vi "Device Connections.vi"(8 "error in":errorcluster, 11 "Class Objects In":T1) -> (0 "error out":errorcluster, 3 "Class Objects Out":T1)   [LabVIEW 2011]
uses:
  Controls/Class Objects.ctl
  Modules/File/Configuration/Configuration.lvclass
  Modules/Hardware/Mass Flow Controller/Mass Flow Controller.lvclass
  Modules/Hardware/Valve Controller/Valve Controller.lvclass
  Modules/Hardware/PID/PID.lvclass
  Modules/Hardware/Power Supply/Power Supply.lvclass
  Modules/Hardware/Multimeter/Multimeter.lvclass
  Modules/Hardware/Vapour Generator/Vapour Generator.lvclass
  Modules/File/TDMS/TDMS.lvclass
  Controls/Detector Type.ctl
  Controls/PS Type.ctl
  Controls/MFC Type.ctl
  Controls/Valve Type.ctl
  Modules/Hardware/Aalborg GFC17/Aalborg GFC17 Connections.ctl
  Controls/Multimeter Type.ctl
  Modules/Hardware/Owlstone GEN-SYS/GEN-SYS Connections.ctl
  Controls/Vapour Generator Type.ctl
  Modules/Hardware/Baseline Mocon piD-Tech plus/Connections.ctl
  Controls/INL PID Connections.ctl
  Modules/Hardware/INL PID/Integrator DAQmx Channels.ctl
  Functional Global Data/Device Params Global.ctl
  Controls/Class Labels.ctl
  Controls/User Interface Action.ctl
  Modules/Hardware/Aalborg GFC17/Aalborg GFC17.lvclass
  Modules/Hardware/Owlstone GEN-SYS/Owlstone GEN-SYS.lvclass
  Modules/Hardware/Baseline Mocon piD-Tech plus/Baseline Mocon piD-Tech plus.lvclass
  Modules/Hardware/INL PID/INL PID.lvclass
panel:
  in  "?":T2(tab)=enum."PID"
  in  "Vapour Generator Type":T3
  in  "Owlstone Gen-SYS":T4={"GEN-SYS VISA resource name"="", "OVG-4"={"Flow Address"=2, "Temp Address"=1}, "OHG-4"={"Flow Address"=2, "Easydew VISA resource name"=""}}
  in  "Vapour Generator Connection":bool caption="Connection"
  in  "INL PID Connections":T5={"PIDs"=1, "Integrator DAQ Channels 1"={"V0"="cDAQ1Mod1/ai0", "S1"="cDAQ1Mod5/port0/line4", "S2"="cDAQ1Mod5/ctr0"}, "Integrator DAQ Channels 2"={"V0"="cDAQ1Mod1/ai0", "S1"="cDAQ1Mod5/port0/line4", "S2"="cDAQ1Mod5/ctr0"}} {"PIDs" min=1 max=2 step=1}
  in  "B-M PID Connections":T7 caption="Baseline-Mocon piD-TECH plus"
  in  "Detector Type":T8 caption="Type"
  in  "Detector Connection":bool=TRUE caption="Connection"
  in  "Power Supply Type":T9 caption="Type"
  in  "Power Supply Connection":bool caption="Connection"
  in  "Power Supply VISA resource name":refnum<visa-resource-name> caption="VISA resource name"
  in  "Multimeter VISA resource name":refnum<visa-resource-name> caption="VISA resource name"
  in  "Multimeter Connection":bool caption="Connection"
  in  "Multimeter Type":T10 caption="Type"
  in  "Aalborg GFC17 Connections":T11={"flow rate setpoint channel"="cDAQ1Mod3/ao0", "flow rate reading channel"="cDAQ1Mod1/ai4", "valve channel"="cDAQ1Mod3/ao1"}
  in  "MFC Type":T12 caption="Type"
  in  "MFC Connection":bool=TRUE caption="Connection"
  in  "Valve Type":T13 caption="Type"
  in  "Valve Connection":bool caption="Connection"
  in  "Valve Controller VISA resource name":refnum<visa-resource-name> caption="VISA resource name"
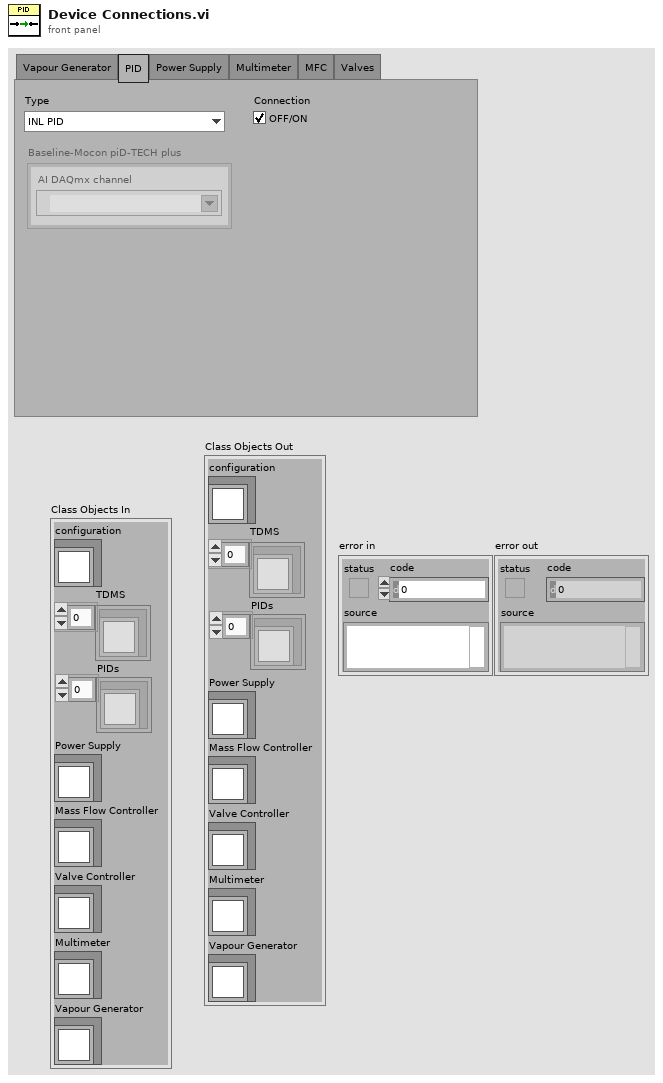
[diagram p1: front panel]
types:
  T1 = typedef "Class Objects.ctl" = cluster{"configuration":refnum<class "Configuration.lvclass">, "TDMS":refnum<class "TDMS.lvclass">[], "Power Supply":refnum<class "Power Supply.lvclass">, "Mass Flow Controller":refnum<class "Mass Flow Controller.lvclass">, "Valve Controller":refnum<class "Valve Controller.lvclass">, "Multimeter":refnum<class "Multimeter.lvclass">, "Vapour Generator":refnum<class "Vapour Generator.lvclass">, "PIDs":refnum<class "PID.lvclass">[]}
  T2 = enum32{"Vapour Generator", "PID", "Power Supply", "Multimeter", "MFC", "Valves"}
  T3 = typedef "Vapour Generator Type.ctl" = enum16{"Owlstone GEN-SYS"}
  T4 = typedef "Owlstone GEN-SYS.lvclass/GEN-SYS Connections.ctl" = cluster{"GEN-SYS VISA resource name":refnum<visa-resource-name>, "OVG-4":cluster{"Flow Address":u8, "Temp Address":u8}, "OHG-4":cluster{"Flow Address":u8, "Easydew VISA resource name":refnum<visa-resource-name>}}
  T5 = typedef "INL PID Connections.ctl" = cluster{"PIDs":u8, "Integrator DAQ Channels 1":T6, "Integrator DAQ Channels 2":T6}
  T6 = typedef "INL PID.lvclass/Integrator DAQmx Channels.ctl" = cluster{"V0":tag, "S1":tag, "S2":tag}
  T7 = typedef "Baseline Mocon piD-Tech plus.lvclass/Connections.ctl" = cluster{"AI DAQmx channel":tag}
  T8 = typedef "Detector Type.ctl" = enum16{"INL PID", "Baseline-Mocon piD-TECH plus"}
  T9 = typedef "PS Type.ctl" = enum16{"Stanford Research PS350", "Keithley 2400"}
  T10 = typedef "Multimeter Type.ctl" = enum16{"Agilent 3458A"}
  T11 = typedef "Aalborg GFC17.lvclass/Aalborg GFC17 Connections.ctl" = cluster{"flow rate setpoint channel":tag, "flow rate reading channel":tag, "valve channel":tag}
  T12 = typedef "MFC Type.ctl" = enum16{"Aalborg GFC17"}
  T13 = typedef "Valve Type.ctl" = enum16{"SMC - INL"}
  T14 = enum8{"Enabled", "Disabled", "Disabled and Grayed Out"}
  T15 = typedef "Device Params Global.ctl" = enum16{"Initialize", "Get Device Settings", "Get Device Connections", "Set Device Settings", "Set Device Connections", "Get All Device Properties"}
  T16 = typedef "Class Labels.ctl" = enum16{"Configuration", "TDMS", "PID", "Power Supply", "Vapour Generator", "MFC", "NMR", "Valve Controller", "Multimeter"}
  T17 = typedef "User Interface Action.ctl" = enum16{"Initialize", "Data Acquisition Disable", "Data View Disable", "Sample Set", "Sample Set 2D Data", "Sample Set x0 & dx", "Sample Add", "Sample Set Cursor", "Sample Set Offset & Multiplier", "Sample Set Axis Labels", "Sample Parameters Disabled", "Sample Parameters Update", "Run Update", "Run Set Offset & Multiplier", "Run Set Axis Labels", "Run Set Cursor", "Run Set Disabled", "Run Parameters Update", "Run Parameters Disabled", "Run Number Set", "Run Number Set Range", "Run Number Set Disabled", "Sample Number Set", "Sample Number Set Range", "Notes Set Value", "Update Plot", "Set Plot Parameters", "Update Concentration Plot", "Time Set", "Clear DAQ Display", "Clear Analysis Display", "Status Bar Set", "Progress Bar Set", "Display Mode Set", "Experiment Type Set", "Analysis Plot Average Set", "Stop"}
  T18 = typedef "Device Connections.ctl" = cluster{"Detector":cluster{"Detector Type":T8, "Connection":bool, "B-M PID":T7, "INL PID Connections":T5}, "Power Supply":cluster{"Type":enum16{"Stanford Research PS350", "Keithley 2400"}, "Connection":bool, "VISA resource name":refnum<visa-resource-name>}, "Mass Flow Controller":cluster{"Type":enum16{"Aalborg GFC17"}, "Connection":bool, "Aalborg GFC17":T11}, "Valve Controller":cluster{"Type":T13, "Connection":bool, "SMC - INL":cluster{"VISA resource name":refnum<visa-resource-name>}}, "Multimeter":cluster{"Multimeter Type":T10, "Connection":bool, "VISA resource name":refnum<visa-resource-name>}, "Vapour Generator":cluster{"Type":T3, "Connection":bool, "Owlstone Gen-SYS":T4}}
  T19 = enum16{"Stanford Research PS350", "Keithley 2400"}
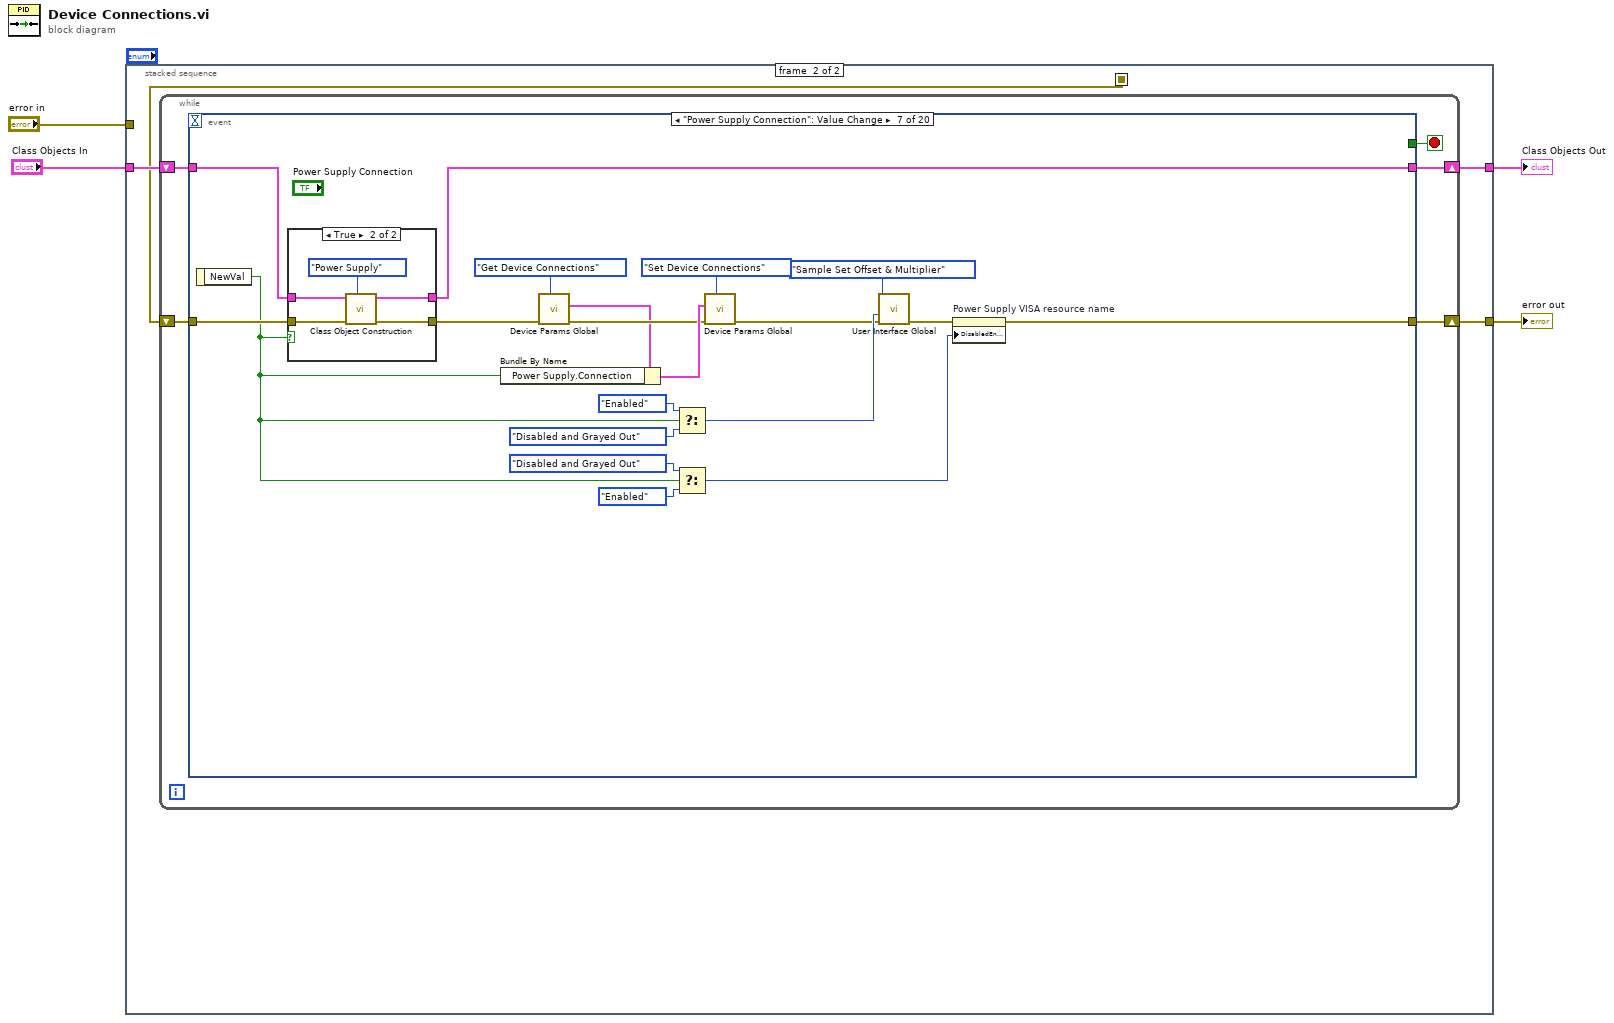
[diagram p0: block diagram]
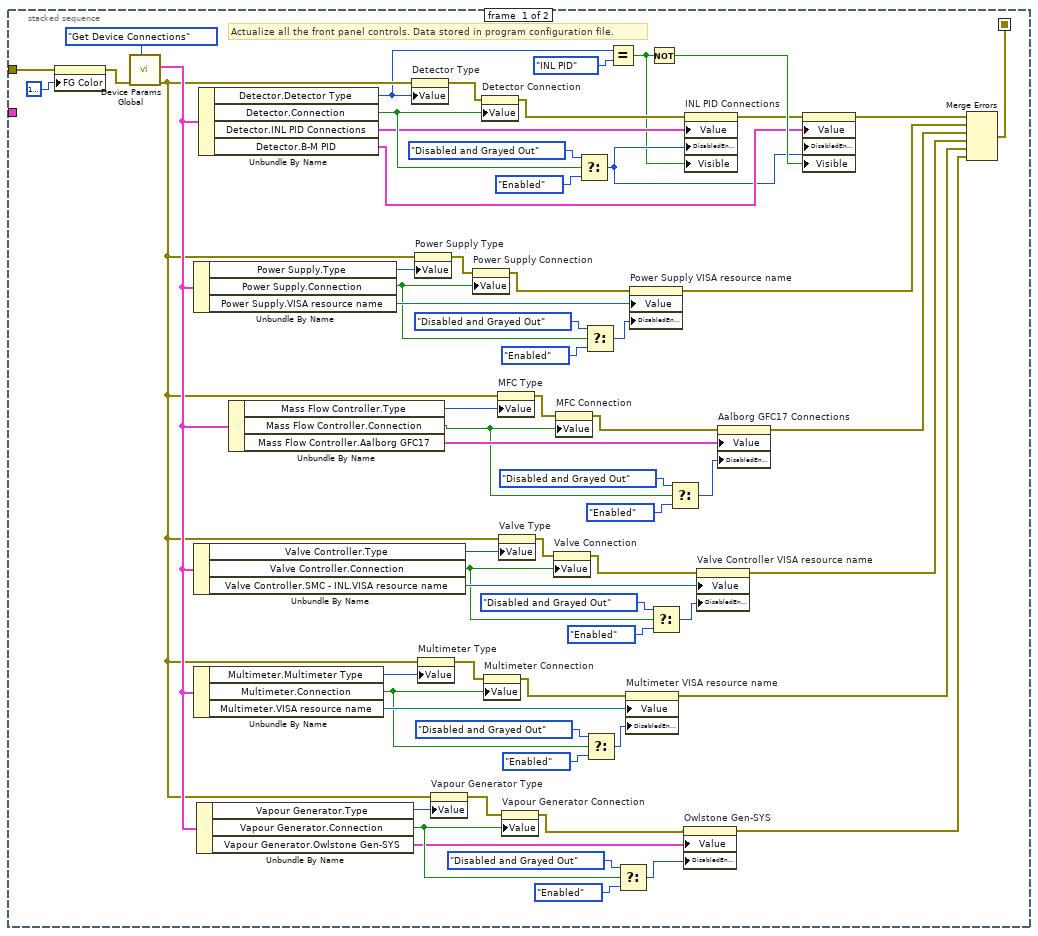
[diagram p2: hidden frame]
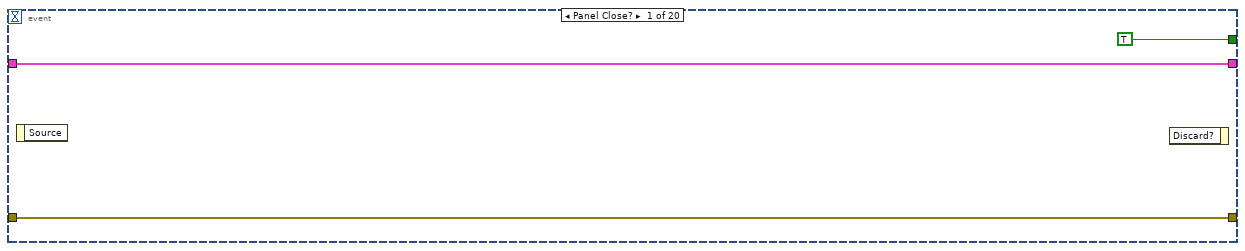
[diagram p3: hidden frame]
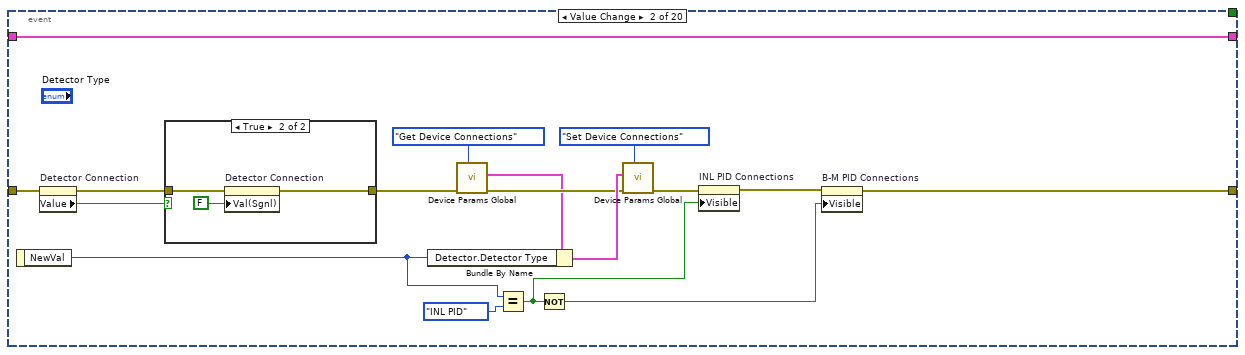
[diagram p4: hidden frame]
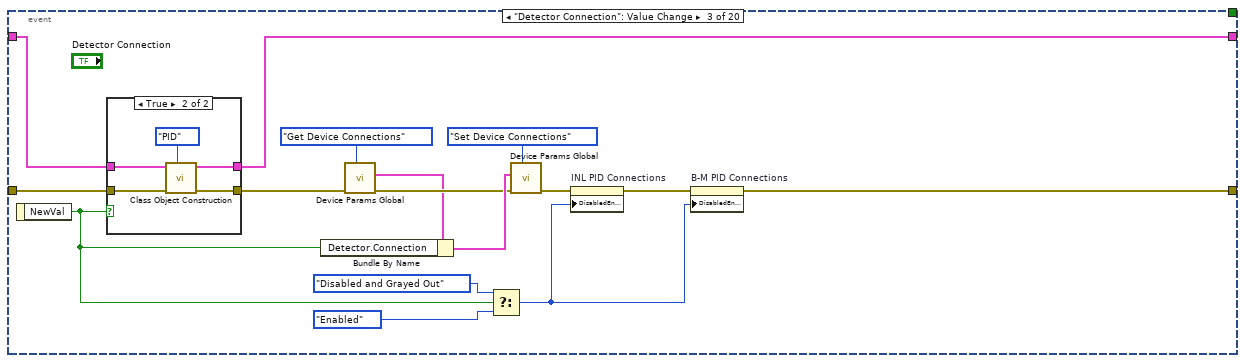
[diagram p6: hidden frame]
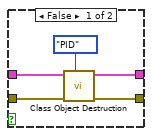
[diagram p7: hidden frame]
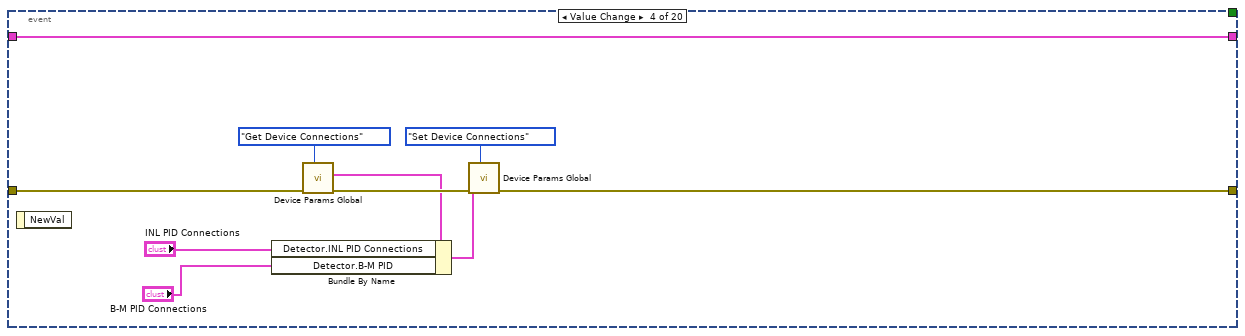
[diagram p8: hidden frame]
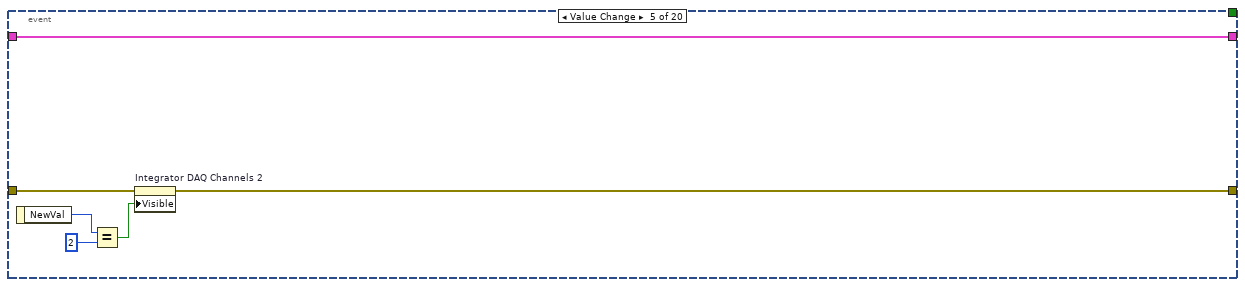
[diagram p9: hidden frame]
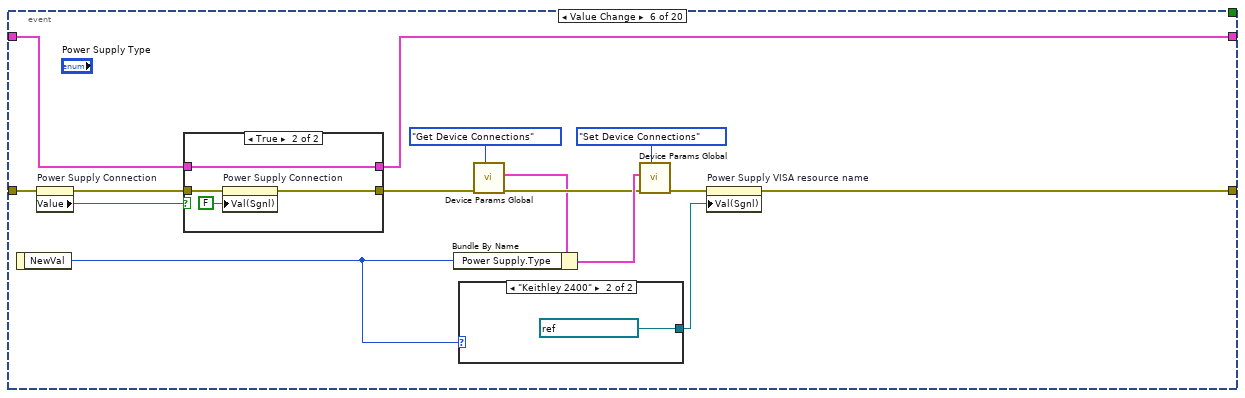
[diagram p10: hidden frame]
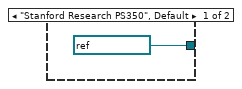
[diagram p11: hidden frame]
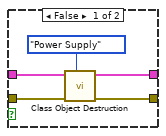
[diagram p13: hidden frame]
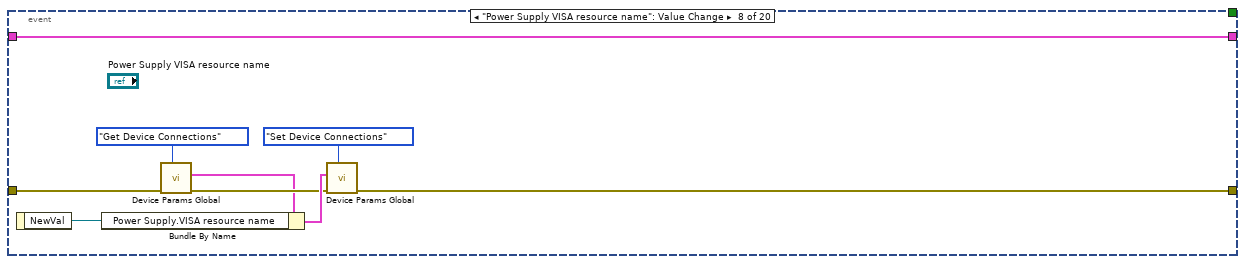
[diagram p14: hidden frame]
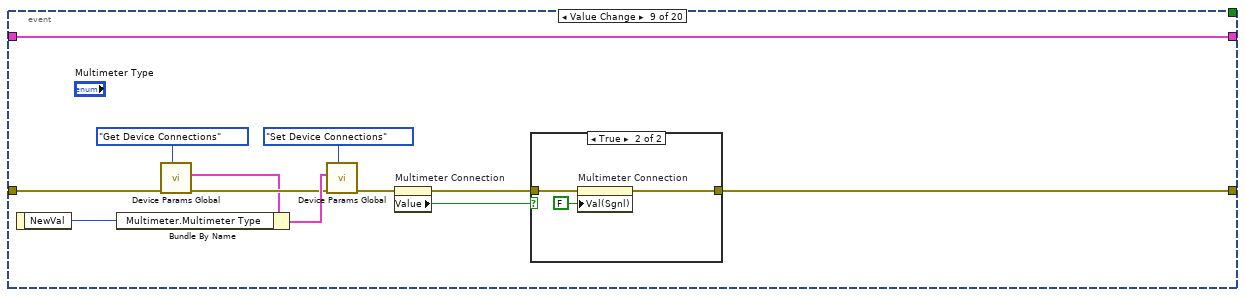
[diagram p15: hidden frame]
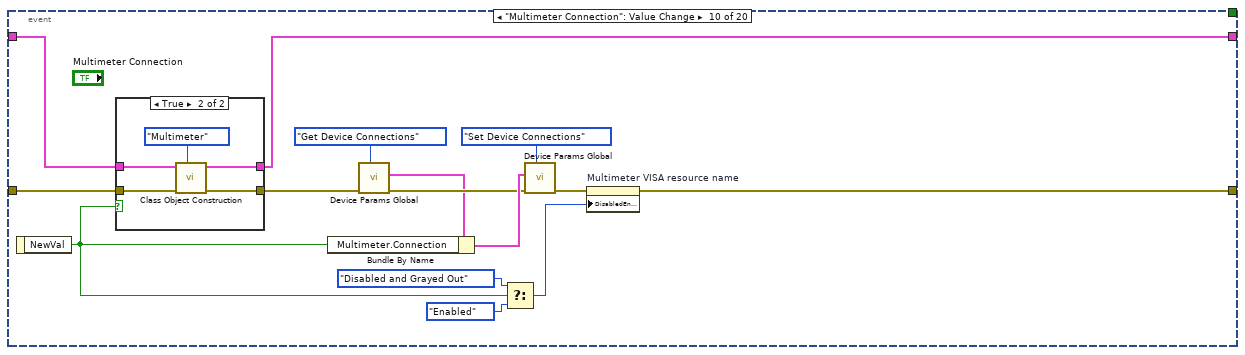
[diagram p17: hidden frame]
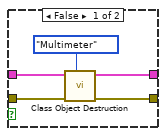
[diagram p18: hidden frame]
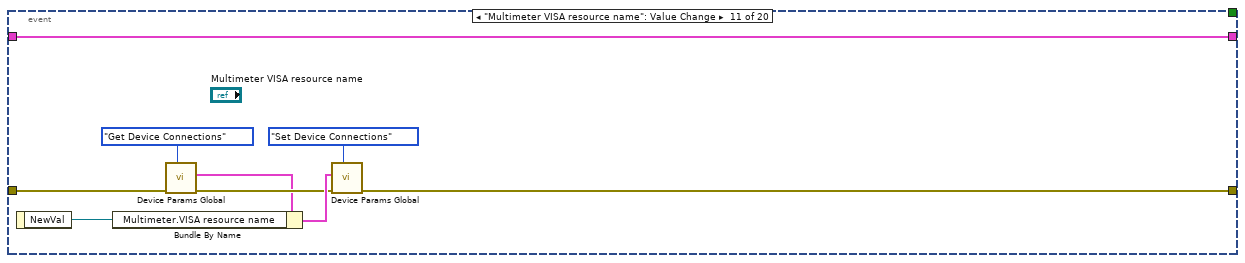
[diagram p19: hidden frame]
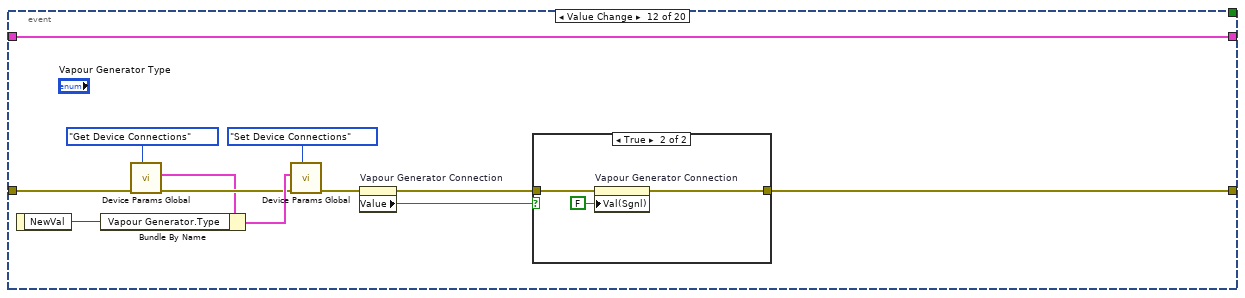
[diagram p20: hidden frame]
diagram:
  n1 = stacked-sequence {
    seq-local: [w35 _] -> [_ w71]
    tunnel: [_ w73] -> w1
    tunnel: "error in" -> [w69 _]
    tunnel: "Class Objects In" -> [_ w72]
    tunnel: [_ w74] -> w2
    frame #0 {
      # "Actualize all the front panel controls. Data stored in program configuration file."
      n2 = property class="TabCtl (strict)"(error in=w69, "FG Color"=u32 16777238) -> (error out=w68:errorcluster)  [unwired: 1 in, 1 out]
      n3 = call "Device Params Global.vi"("action"=Device_Params_Global."Get Device Connections", "error in"=w68) -> ("error out"=w16:errorcluster, "Device Connections OUT"=w25:T18)  [unwired: 7 in, 1 out]
      n4 = Unbundle By Name(w25) -> ("Power Supply.Type"=w63:T19, "Power Supply.Connection"=w46:bool, "Power Supply.VISA resource name"=w62:refnum<visa-resource-name>)
      n5 = Unbundle By Name(w25) -> ("Valve Controller.Type"=w57:T13, "Valve Controller.Connection"=w38:bool, "Valve Controller.SMC - INL.VISA resource name"=w54:refnum<visa-resource-name>)
      n6 = Unbundle By Name(w25) -> ("Multimeter.Multimeter Type"=w34:T10, "Multimeter.Connection"=w27:bool, "Multimeter.VISA resource name"=w31:refnum<visa-resource-name>)
      n7 = Unbundle By Name(w25) -> ("Vapour Generator.Type"=w15:T3, "Vapour Generator.Connection"=w22:bool, "Vapour Generator.Owlstone Gen-SYS"=w18:T4)
      n8 = Unbundle By Name(w25) -> ("Detector.Detector Type"=w12:T8, "Detector.Connection"=w50:bool, "Detector.INL PID Connections"=w7:T5, "Detector.B-M PID"=w10:T7)
      n9 = Unbundle By Name(w25) -> ("Mass Flow Controller.Type"=w61:enum16{"Aalborg GFC17"}, "Mass Flow Controller.Connection"=w42:bool, "Mass Flow Controller.Aalborg GFC17"=w58:T11)
      n10 = property on="Detector Type" class="Enum (strict)"(error in=w16, "Value"=w12) -> (error out=w66:errorcluster)  [unwired: 1 in, 1 out]
      n11 = property on="Power Supply Type" class="Enum (strict)"(error in=w16, "Value"=w63) -> (error out=w65:errorcluster)  [unwired: 1 in, 1 out]
      n12 = property on="Multimeter Type" class="Enum (strict)"(error in=w16, "Value"=w34) -> (error out=w33:errorcluster)  [unwired: 1 in, 1 out]
      n13 = property on="Vapour Generator Type" class="Enum (strict)"(error in=w16, "Value"=w15) -> (error out=w17:errorcluster)  [unwired: 1 in, 1 out]
      n14 = property on="Power Supply Connection" class="Bool (strict)"(error in=w65, "Value"=w46) -> (error out=w64:errorcluster)  [unwired: 1 in, 1 out]
      n15 = property on="Detector Connection" class="Bool (strict)"(error in=w66, "Value"=w50) -> (error out=w9:errorcluster)  [unwired: 1 in, 1 out]
      n16 = property on="Multimeter Connection" class="Bool (strict)"(error in=w33, "Value"=w27) -> (error out=w30:errorcluster)  [unwired: 1 in, 1 out]
      n17 = property on="MFC Type" class="Enum (strict)"(error in=w16, "Value"=w61) -> (error out=w60:errorcluster)  [unwired: 1 in, 1 out]
      n18 = property on="Valve Type" class="Enum (strict)"(error in=w16, "Value"=w57) -> (error out=w56:errorcluster)  [unwired: 1 in, 1 out]
      n19 = property on="Vapour Generator Connection" class="Bool (strict)"(error in=w17, "Value"=w22) -> (error out=w19:errorcluster)  [unwired: 1 in, 1 out]
      n20 = property on="Valve Connection" class="Bool (strict)"(error in=w56, "Value"=w38) -> (error out=w55:errorcluster)  [unwired: 1 in, 1 out]
      n21 = property on="MFC Connection" class="Bool (strict)"(error in=w60, "Value"=w42) -> (error out=w59:errorcluster)  [unwired: 1 in, 1 out]
      n22 = Select(t=T14."Disabled and Grayed Out" ("Disabled"), s=w50, f=T14."Enabled") -> (s? t:f=w6:T14)
      n23 = Select(t=T14."Disabled and Grayed Out" ("Disabled"), s=w46, f=T14."Enabled") -> (s? t:f=w45:T14)
      n24 = Select(t=T14."Disabled and Grayed Out" ("Disabled"), s=w27, f=T14."Enabled") -> (s? t:f=w29:T14)
      n25 = Equal?(x=w12, y=Detector_Type."INL PID" ("Detector.Detector Type")) -> (x = y?=w5:bool)
      n26 = Select(t=T14."Disabled and Grayed Out" ("Disabled"), s=w22, f=T14."Enabled") -> (s? t:f=w21:T14)
      n27 = property on="Multimeter VISA resource name" class="VISAName"(error in=w30, "Value"=w31, "DisabledEnum"=w29) -> (error out=w26:errorcluster)  [unwired: 1 in, 1 out]
      n28 = property on="Power Supply VISA resource name" class="VISAName"(error in=w64, "Value"=w62, "DisabledEnum"=w45) -> (error out=w53:errorcluster)  [unwired: 1 in, 1 out]
      n29 = Not(x=w5) -> (.not. x?=w11:bool)
      n30 = Select(t=T14."Disabled and Grayed Out" ("Disabled"), s=w38, f=T14."Enabled") -> (s? t:f=w37:T14)
      n31 = Select(t=T14."Disabled and Grayed Out" ("Disabled"), s=w42, f=T14."Enabled") -> (s? t:f=w41:T14)
      n32 = property on="Owlstone Gen-SYS" class="Clust (strict)"(error in=w19, "Value"=w18, "DisabledEnum"=w21) -> (error out=w20:errorcluster)  [unwired: 1 in, 1 out]
      n33 = property on="INL PID Connections" class="Clust (strict)"(error in=w9, "Value"=w7, "DisabledEnum"=w6, "Visible"=w5) -> (error out=w8:errorcluster)  [unwired: 1 in, 1 out]
      n34 = property on="Valve Controller VISA resource name" class="VISAName"(error in=w55, "Value"=w54, "DisabledEnum"=w37) -> (error out=w36:errorcluster)  [unwired: 1 in, 1 out]
      n35 = property on="Aalborg GFC17 Connections" class="Clust (strict)"(error in=w59, "Value"=w58, "DisabledEnum"=w41) -> (error out=w52:errorcluster)  [unwired: 1 in, 1 out]
      n36 = property on="B-M PID Connections" class="Clust (strict)"(error in=w8, "Value"=w10, "DisabledEnum"=w6, "Visible"=w11) -> (error out=w14:errorcluster)  [unwired: 1 in, 1 out]
      n37 = Merge Errors(w14, w53, w52, w36, w26, w20) -> (w35:errorcluster)
    }
    frame #1 {
      n38 = while {
        shift-right: [w77] -> w74
        shift-left: w72 -> [w78]
        shift-right: [w75] -> w73
        shift-left: w71 -> [w76]
        stop <- w79 stop-if-true
        n39 = event shown="[6] \"Power Supply Connection\": Value Change" {
          selector: _ -> [_ _ _ _ _ _ _ _ _ _ _ _ _ _ _ _ _ _ _ _]
          dyn-events: _ -> [_ _ _ _ _ _ _ _ _ _ _ _ _ _ _ _ _ _ _ _]
          timeout: _ -> [_ _ _ _ _ _ _ _ _ _ _ _ _ _ _ _ _ _ _ _]
          tunnel: [w81 w86 w107 w132 w140 w154 w183 w205 w208 w230 w250 w259 w274 w301 w316 w335 w349 w366 w381 w397] -> w75
          tunnel: [TRUE ("Discard?") _ _ _ _ _ _ _ _ _ _ _ _ _ _ _ _ _ _ _] -> w79
          tunnel: w78 -> [w82 w99 w119 w139 w143 w160 w188 w203 w219 w228 w249 w258 w288 w300 w319 w338 w357 w369 w387 w405]
          tunnel: [w82 w99 w118 w139 w143 w156 w187 w203 w219 w227 w249 w258 w277 w300 w319 w337 w357 w369 w386 w405] -> w77
          tunnel: w76 -> [w81 w98 w117 w133 w141 w159 w177 w201 w213 w229 w252 w264 w287 w302 w310 w336 w351 w360 w385 w399]
          event Panel Close? {
            n40 = event-data() -> ()  [unwired: 1 in, 1 out]
            n41 = event-data() -> ()  [unwired: 2 in, 1 out]
          }
          event Value Change {
            n42 = event-data() -> ("NewVal"=w88:T8)  [unwired: 1 in]
            n43 = property on="Detector Connection" class="Bool (strict)"(error in=w98) -> (error out=w96:errorcluster, "Value"=w97:bool)  [unwired: 1 in, 1 out]
            n44 = case shown="True" w97 {
              tunnel: w96 -> [w100 w103]
              tunnel: [w100 w102] -> w90
              frame False {
              }
              frame True {
                n45 = property on="Detector Connection" class="Bool (strict)"(error in=w103, "Val(Sgnl)"=FALSE ("Detector Connection")) -> (error out=w102:errorcluster)  [unwired: 1 in, 1 out]
              }
            }
            n46 = call "Device Params Global.vi"("action"=Device_Params_Global."Get Device Connections", "error in"=w90) -> ("error out"=w92:errorcluster, "Device Connections OUT"=w91:T18)  [unwired: 7 in, 1 out]
            n47 = Bundle By Name(cluster=w91, "Detector.Detector Type"=w88) -> (w94:T18)
            n48 = Equal?(x=w88, y=Detector_Type."INL PID" ("Detector.Detector Type")) -> (x = y?=w84:bool)
            n49 = Not(x=w84) -> (.not. x?=w87:bool)
            n50 = call "Device Params Global.vi"("action"=Device_Params_Global."Set Device Connections", "error in"=w92, "Device Connections IN"=w94) -> ("error out"=w85:errorcluster)  [unwired: 6 in, 2 out]
            n51 = property on="INL PID Connections" class="Clust (strict)"(error in=w85, "Visible"=w84) -> (error out=w83:errorcluster)  [unwired: 1 in, 1 out]
            n52 = property on="B-M PID Connections" class="Clust (strict)"(error in=w83, "Visible"=w87) -> (error out=w86:errorcluster)  [unwired: 1 in, 1 out]
          }
          event "Detector Connection": Value Change {
            n53 = event-data() -> ("NewVal"=w108:bool)  [unwired: 1 in]
            n54 = case shown="True" w108 {
              tunnel: w119 -> [w122 w129]
              tunnel: w117 -> [w124 w127]
              tunnel: [w121 w126] -> w118
              tunnel: [w123 w125] -> w109
              frame False {
                n55 = call "Class Object Destruction.vi"("class labels"=Class_Labels."PID", "error in"=w124, "classes in"=w122) -> ("error out"=w123:errorcluster, "classes out"=w121:T1)  [unwired: 7 in]
              }
              frame True {
                n56 = call "Class Object Construction.vi"("class"=Class_Labels."PID", "error in"=w127, "classes in"=w129) -> ("error out"=w125:errorcluster, "classes out"=w126:T1)  [unwired: 6 in]
              }
            }
            n57 = call "Device Params Global.vi"("action"=Device_Params_Global."Get Device Connections", "error in"=w109) -> ("error out"=w111:errorcluster, "Device Connections OUT"=w110:T18)  [unwired: 7 in, 1 out]
            n58 = Bundle By Name(cluster=w110, "Detector.Connection"=w108) -> (w113:T18)
            n59 = Select(t=T14."Disabled and Grayed Out" ("Disabled"), s=w108, f=T14."Enabled" ("Disabled")) -> (s? t:f=w105:T14)
            n60 = call "Device Params Global.vi"("action"=Device_Params_Global."Set Device Connections", "error in"=w111, "Device Connections IN"=w113) -> ("error out"=w106:errorcluster)  [unwired: 6 in, 2 out]
            n61 = property on="INL PID Connections" class="Clust (strict)"(error in=w106, "DisabledEnum"=w105) -> (error out=w104:errorcluster)  [unwired: 1 in, 1 out]
            n62 = property on="B-M PID Connections" class="Clust (strict)"(error in=w104, "DisabledEnum"=w105) -> (error out=w107:errorcluster)  [unwired: 1 in, 1 out]
          }
          event Value Change {
            n63 = event-data() -> ()  [unwired: 1 in, 1 out]
            n64 = call "Device Params Global.vi"("action"=Device_Params_Global."Get Device Connections", "error in"=w133) -> ("error out"=w135:errorcluster, "Device Connections OUT"=w134:T18)  [unwired: 7 in, 1 out]
            n65 = Bundle By Name(cluster=w134, "Detector.INL PID Connections"="INL PID Connections", "Detector.B-M PID"="B-M PID Connections") -> (w137:T18)
            n66 = call "Device Params Global.vi"("action"=Device_Params_Global."Set Device Connections", "error in"=w135, "Device Connections IN"=w137) -> ("error out"=w132:errorcluster)  [unwired: 6 in, 2 out]
          }
          event Value Change {
            n67 = event-data() -> ("NewVal"=w144:u8)  [unwired: 1 in]
            n68 = Equal?(x=w144, y=2) -> (x = y?=w142:bool)
            n69 = property on="Integrator DAQ Channels 2" class="Clust (strict)"(error in=w141, "Visible"=w142) -> (error out=w140:errorcluster)  [unwired: 1 in, 1 out]
          }
          event Value Change {
            n70 = event-data() -> ("NewVal"=w146:T9)  [unwired: 1 in]
            n71 = property on="Power Supply Connection" class="Bool (strict)"(error in=w159) -> (error out=w158:errorcluster, "Value"=w157:bool)  [unwired: 1 in, 1 out]
            n72 = case shown="True" w157 {
              tunnel: w160 -> [w164 w166]
              tunnel: [w163 w167] -> w148
              tunnel: [w164 w166] -> w156
              tunnel: w158 -> [w163 w165]
              frame False {
              }
              frame True {
                n73 = property on="Power Supply Connection" class="Bool (strict)"(error in=w165, "Val(Sgnl)"=FALSE ("PS Connection")) -> (error out=w167:errorcluster)  [unwired: 1 in, 1 out]
              }
            }
            n74 = case shown="\"Keithley 2400\"" w146 {
              tunnel: [refnum<visa-resource-name> "SR_PS350" ("VISA resource name") refnum<visa-resource-name> "Keithley_2400" ("VISA resource name")] -> w155
              frame "Stanford Research PS350", Default {
              }
              frame "Keithley 2400" {
              }
            }
            n75 = call "Device Params Global.vi"("action"=Device_Params_Global."Get Device Connections", "error in"=w148) -> ("error out"=w150:errorcluster, "Device Connections OUT"=w149:T18)  [unwired: 7 in, 1 out]
            n76 = Bundle By Name(cluster=w149, "Power Supply.Type"=w146) -> (w152:T18)
            n77 = call "Device Params Global.vi"("action"=Device_Params_Global."Set Device Connections", "error in"=w150, "Device Connections IN"=w152) -> ("error out"=w147:errorcluster)  [unwired: 6 in, 2 out]
            n78 = property on="Power Supply VISA resource name" class="VISAName"(error in=w147, "Val(Sgnl)"=w155) -> (error out=w154:errorcluster)  [unwired: 1 in, 1 out]
          }
          event "Power Supply Connection": Value Change {
            n79 = event-data() -> ("NewVal"=w169:bool)  [unwired: 1 in]
            n80 = case shown="True" w169 {
              tunnel: w188 -> [w192 w198]
              tunnel: [w191 w195] -> w187
              tunnel: [w193 w196] -> w171
              tunnel: w177 -> [w189 w197]
              frame False {
                n81 = call "Class Object Destruction.vi"("class labels"=Class_Labels."Power Supply", "error in"=w189, "classes in"=w192) -> ("error out"=w193:errorcluster, "classes out"=w191:T1)  [unwired: 7 in]
              }
              frame True {
                n82 = call "Class Object Construction.vi"("class"=Class_Labels."Power Supply", "error in"=w197, "classes in"=w198) -> ("error out"=w196:errorcluster, "classes out"=w195:T1)  [unwired: 6 in]
              }
            }
            n83 = call "Device Params Global.vi"("action"=Device_Params_Global."Get Device Connections", "error in"=w171) -> ("error out"=w173:errorcluster, "Device Connections OUT"=w172:T18)  [unwired: 7 in, 1 out]
            n84 = Bundle By Name(cluster=w172, "Power Supply.Connection"=w169) -> (w175:T18)
            n85 = Select(t=T14."Enabled" ("Disabled"), s=w169, f=T14."Disabled and Grayed Out" ("Disabled")) -> (s? t:f=w178:T14)
            n86 = Select(t=T14."Disabled and Grayed Out" ("Disabled"), s=w169, f=T14."Enabled" ("Disabled")) -> (s? t:f=w182:T14)
            n87 = call "Device Params Global.vi"("action"=Device_Params_Global."Set Device Connections", "error in"=w173, "Device Connections IN"=w175) -> ("error out"=w170:errorcluster)  [unwired: 6 in, 2 out]
            n88 = call "User Interface Global.vi"("error in"=w170, "data1"=w178, "action"=User_Interface_Action."Sample Set Offset & Multiplier") -> ("error out"=w184:errorcluster)  [unwired: 8 in]
            n89 = property on="Power Supply VISA resource name" class="VISAName"(error in=w184, "DisabledEnum"=w182) -> (error out=w183:errorcluster)  [unwired: 1 in, 1 out]
          }
          event "Power Supply VISA resource name": Value Change {
            n90 = event-data() -> ("NewVal"=w204:refnum<visa-resource-name>)  [unwired: 1 in]
            n91 = call "Device Params Global.vi"("action"=Device_Params_Global."Get Device Connections", "error in"=w201) -> ("error out"=w200:errorcluster, "Device Connections OUT"=w199:T18)  [unwired: 7 in, 1 out]
            n92 = Bundle By Name(cluster=w199, "Power Supply.VISA resource name"=w204) -> (w206:T18)
            n93 = call "Device Params Global.vi"("action"=Device_Params_Global."Set Device Connections", "error in"=w200, "Device Connections IN"=w206) -> ("error out"=w205:errorcluster)  [unwired: 6 in, 2 out]
          }
          event Value Change {
            n94 = event-data() -> ("NewVal"=w212:T10)  [unwired: 1 in]
            n95 = call "Device Params Global.vi"("action"=Device_Params_Global."Get Device Connections", "error in"=w213) -> ("error out"=w215:errorcluster, "Device Connections OUT"=w214:T18)  [unwired: 7 in, 1 out]
            n96 = Bundle By Name(cluster=w214, "Multimeter.Multimeter Type"=w212) -> (w217:T18)
            n97 = call "Device Params Global.vi"("action"=Device_Params_Global."Set Device Connections", "error in"=w215, "Device Connections IN"=w217) -> ("error out"=w211:errorcluster)  [unwired: 6 in, 2 out]
            n98 = property on="Multimeter Connection" class="Bool (strict)"(error in=w211) -> (error out=w209:errorcluster, "Value"=w210:bool)  [unwired: 1 in, 1 out]
            n99 = case shown="True" w210 {
              tunnel: w209 -> [w220 w223]
              tunnel: [w220 w221] -> w208
              frame False {
              }
              frame True {
                n100 = property on="Multimeter Connection" class="Bool (strict)"(error in=w223, "Val(Sgnl)"=FALSE ("Value (Signaling)")) -> (error out=w221:errorcluster)  [unwired: 1 in, 1 out]
              }
            }
          }
          event "Multimeter Connection": Value Change {
            n101 = event-data() -> ("NewVal"=w226:bool)  [unwired: 1 in]
            n102 = case shown="True" w226 {
              tunnel: w228 -> [w242 w248]
              tunnel: [w241 w246] -> w227
              tunnel: [w243 w245] -> w225
              tunnel: w229 -> [w239 w244]
              frame False {
                n103 = call "Class Object Destruction.vi"("class labels"=Class_Labels."Multimeter", "error in"=w239, "classes in"=w242) -> ("error out"=w243:errorcluster, "classes out"=w241:T1)  [unwired: 7 in]
              }
              frame True {
                n104 = call "Class Object Construction.vi"("class"=Class_Labels."Multimeter", "error in"=w244, "classes in"=w248) -> ("error out"=w245:errorcluster, "classes out"=w246:T1)  [unwired: 6 in]
              }
            }
            n105 = call "Device Params Global.vi"("action"=Device_Params_Global."Get Device Connections", "error in"=w225) -> ("error out"=w235:errorcluster, "Device Connections OUT"=w234:T18)  [unwired: 7 in, 1 out]
            n106 = Bundle By Name(cluster=w234, "Multimeter.Connection"=w226) -> (w237:T18)
            n107 = Select(t=T14."Disabled and Grayed Out" ("Disabled"), s=w226, f=T14."Enabled" ("Disabled")) -> (s? t:f=w231:T14)
            n108 = call "Device Params Global.vi"("action"=Device_Params_Global."Set Device Connections", "error in"=w235, "Device Connections IN"=w237) -> ("error out"=w232:errorcluster)  [unwired: 6 in, 2 out]
            n109 = property on="Multimeter VISA resource name" class="VISAName"(error in=w232, "DisabledEnum"=w231) -> (error out=w230:errorcluster)  [unwired: 1 in, 1 out]
          }
          event "Multimeter VISA resource name": Value Change {
            n110 = event-data() -> ("NewVal"=w251:refnum<visa-resource-name>)  [unwired: 1 in]
            n111 = call "Device Params Global.vi"("action"=Device_Params_Global."Get Device Connections", "error in"=w252) -> ("error out"=w254:errorcluster, "Device Connections OUT"=w253:T18)  [unwired: 7 in, 1 out]
            n112 = Bundle By Name(cluster=w253, "Multimeter.VISA resource name"=w251) -> (w256:T18)
            n113 = call "Device Params Global.vi"("action"=Device_Params_Global."Set Device Connections", "error in"=w254, "Device Connections IN"=w256) -> ("error out"=w250:errorcluster)  [unwired: 6 in, 2 out]
          }
          event Value Change {
            n114 = event-data() -> ("NewVal"=w263:T3)  [unwired: 1 in]
            n115 = call "Device Params Global.vi"("action"=Device_Params_Global."Get Device Connections", "error in"=w264) -> ("error out"=w266:errorcluster, "Device Connections OUT"=w265:T18)  [unwired: 7 in, 1 out]
            n116 = Bundle By Name(cluster=w265, "Vapour Generator.Type"=w263) -> (w268:T18)
            n117 = call "Device Params Global.vi"("action"=Device_Params_Global."Set Device Connections", "error in"=w266, "Device Connections IN"=w268) -> ("error out"=w262:errorcluster)  [unwired: 6 in, 2 out]
            n118 = property on="Vapour Generator Connection" class="Bool (strict)"(error in=w262) -> (error out=w260:errorcluster, "Value"=w261:bool)  [unwired: 1 in, 1 out]
            n119 = case shown="True" w261 {
              tunnel: w260 -> [w270 w273]
              tunnel: [w270 w271] -> w259
              frame False {
              }
              frame True {
                n120 = property on="Vapour Generator Connection" class="Bool (strict)"(error in=w273, "Val(Sgnl)"=FALSE ("Value (Signaling)")) -> (error out=w271:errorcluster)  [unwired: 1 in, 1 out]
              }
            }
          }
          event "Vapour Generator Connection": Value Change {
            n121 = event-data() -> ("NewVal"=w279:bool)  [unwired: 1 in]
            n122 = case shown="True" w279 {
              tunnel: w288 -> [w291 w298]
              tunnel: w287 -> [w293 w296]
              tunnel: [w290 w295] -> w277
              tunnel: [w292 w294] -> w282
              frame False {
                n123 = call "Class Object Destruction.vi"("class labels"=Class_Labels."Vapour Generator", "error in"=w293, "classes in"=w291) -> ("error out"=w292:errorcluster, "classes out"=w290:T1)  [unwired: 7 in]
              }
              frame True {
                n124 = call "Class Object Construction.vi"("class"=Class_Labels."Vapour Generator", "error in"=w296, "classes in"=w298) -> ("error out"=w294:errorcluster, "classes out"=w295:T1)  [unwired: 6 in]
              }
            }
            n125 = call "Device Params Global.vi"("action"=Device_Params_Global."Get Device Connections", "error in"=w282) -> ("error out"=w285:errorcluster, "Device Connections OUT"=w286:T18)  [unwired: 7 in, 1 out]
            n126 = Bundle By Name(cluster=w286, "Vapour Generator.Connection"=w279) -> (w283:T18)
            n127 = Select(t=T14."Disabled and Grayed Out" ("Disabled"), s=w279, f=T14."Enabled" ("Disabled")) -> (s? t:f=w275:T14)
            n128 = call "Device Params Global.vi"("action"=Device_Params_Global."Set Device Connections", "error in"=w285, "Device Connections IN"=w283) -> ("error out"=w276:errorcluster)  [unwired: 6 in, 2 out]
            n129 = property on="Owlstone Gen-SYS" class="Clust (strict)"(error in=w276, "DisabledEnum"=w275) -> (error out=w274:errorcluster)  [unwired: 1 in, 1 out]
          }
          event Value Change {
            n130 = event-data() -> ("NewVal"=w299:T4)  [unwired: 1 in]
            n131 = call "Device Params Global.vi"("action"=Device_Params_Global."Get Device Connections", "error in"=w302) -> ("error out"=w304:errorcluster, "Device Connections OUT"=w303:T18)  [unwired: 7 in, 1 out]
            n132 = Bundle By Name(cluster=w303, "Vapour Generator.Owlstone Gen-SYS"=w299) -> (w306:T18)
            n133 = call "Device Params Global.vi"("action"=Device_Params_Global."Set Device Connections", "error in"=w304, "Device Connections IN"=w306) -> ("error out"=w301:errorcluster)  [unwired: 6 in, 2 out]
          }
          event Value Change {
            n134 = event-data() -> ("NewVal"=w308:T12)  [unwired: 1 in]
            n135 = call "Device Params Global.vi"("action"=Device_Params_Global."Get Device Connections", "error in"=w310) -> ("error out"=w312:errorcluster, "Device Connections OUT"=w311:T18)  [unwired: 7 in, 1 out]
            n136 = Bundle By Name(cluster=w311, "Mass Flow Controller.Type"=w308) -> (w314:T18)
            n137 = call "Device Params Global.vi"("action"=Device_Params_Global."Set Device Connections", "error in"=w312, "Device Connections IN"=w314) -> ("error out"=w309:errorcluster)  [unwired: 6 in, 2 out]
            n138 = property on="MFC Connection" class="Bool (strict)"(error in=w309) -> (error out=w317:errorcluster, "Value"=w318:bool)  [unwired: 1 in, 1 out]
            n139 = case shown="True" w318 {
              tunnel: w317 -> [w320 w323]
              tunnel: [w320 w321] -> w316
              frame False {
              }
              frame True {
                n140 = property on="MFC Connection" class="Bool (strict)"(error in=w323, "Val(Sgnl)"=FALSE ("Value (Signaling)")) -> (error out=w321:errorcluster)  [unwired: 1 in, 1 out]
              }
            }
          }
          event "MFC Connection": Value Change {
            n141 = event-data() -> ("NewVal"=w325:bool)  [unwired: 1 in]
            n142 = case shown="False" w325 {
              tunnel: w338 -> [w341 w348]
              tunnel: w336 -> [w343 w346]
              tunnel: [w340 w345] -> w337
              tunnel: [w342 w344] -> w326
              frame False {
                n143 = call "Class Object Destruction.vi"("class labels"=Class_Labels."MFC", "error in"=w343, "classes in"=w341) -> ("error out"=w342:errorcluster, "classes out"=w340:T1)  [unwired: 7 in]
              }
              frame True {
                n144 = call "Class Object Construction.vi"("class"=Class_Labels."MFC", "error in"=w346, "classes in"=w348) -> ("error out"=w344:errorcluster, "classes out"=w345:T1)  [unwired: 6 in]
              }
            }
            n145 = call "Device Params Global.vi"("action"=Device_Params_Global."Get Device Connections", "error in"=w326) -> ("error out"=w328:errorcluster, "Device Connections OUT"=w327:T18)  [unwired: 7 in, 1 out]
            n146 = Bundle By Name(cluster=w327, "Mass Flow Controller.Connection"=w325) -> (w330:T18)
            n147 = Select(t=T14."Disabled and Grayed Out" ("Disabled"), s=w325, f=T14."Enabled" ("Disabled")) -> (s? t:f=w332:T14)
            n148 = call "Device Params Global.vi"("action"=Device_Params_Global."Set Device Connections", "error in"=w328, "Device Connections IN"=w330) -> ("error out"=w324:errorcluster)  [unwired: 6 in, 2 out]
            n149 = property on="Aalborg GFC17 Connections" class="Clust (strict)"(error in=w324, "DisabledEnum"=w332) -> (error out=w335:errorcluster)  [unwired: 1 in, 1 out]
          }
          event Value Change {
            n150 = event-data() -> ("NewVal"=w350:T11)  [unwired: 1 in]
            n151 = call "Device Params Global.vi"("action"=Device_Params_Global."Get Device Connections", "error in"=w351) -> ("error out"=w353:errorcluster, "Device Connections OUT"=w352:T18)  [unwired: 7 in, 1 out]
            n152 = Bundle By Name(cluster=w352, "Mass Flow Controller.Aalborg GFC17"=w350) -> (w355:T18)
            n153 = call "Device Params Global.vi"("action"=Device_Params_Global."Set Device Connections", "error in"=w353, "Device Connections IN"=w355) -> ("error out"=w349:errorcluster)  [unwired: 6 in, 2 out]
          }
          event Value Change {
            n154 = event-data() -> ("NewVal"=w358:T13)  [unwired: 1 in]
            n155 = call "Device Params Global.vi"("action"=Device_Params_Global."Get Device Connections", "error in"=w360) -> ("error out"=w362:errorcluster, "Device Connections OUT"=w361:T18)  [unwired: 7 in, 1 out]
            n156 = Bundle By Name(cluster=w361, "Valve Controller.Type"=w358) -> (w364:T18)
            n157 = call "Device Params Global.vi"("action"=Device_Params_Global."Set Device Connections", "error in"=w362, "Device Connections IN"=w364) -> ("error out"=w359:errorcluster)  [unwired: 6 in, 2 out]
            n158 = property on="Valve Connection" class="Bool (strict)"(error in=w359) -> (error out=w368:errorcluster, "Value"=w367:bool)  [unwired: 1 in, 1 out]
            n159 = case shown="True" w367 {
              tunnel: w368 -> [w370 w373]
              tunnel: [w370 w371] -> w366
              frame False {
              }
              frame True {
                n160 = property on="Valve Connection" class="Bool (strict)"(error in=w373, "Val(Sgnl)"=FALSE ("Value (Signaling)")) -> (error out=w371:errorcluster)  [unwired: 1 in, 1 out]
              }
            }
          }
          event "Valve Connection": Value Change {
            n161 = event-data() -> ("NewVal"=w374:bool)  [unwired: 1 in]
            n162 = case shown="True" w374 {
              tunnel: w387 -> [w390 w396]
              tunnel: [w389 w394] -> w386
              tunnel: [w391 w393] -> w375
              tunnel: w385 -> [_ w392]
              frame False {
                n163 = call "Class Object Destruction.vi"("class labels"=Class_Labels."Valve Controller", "classes in"=w390) -> ("error out"=w391:errorcluster, "classes out"=w389:T1)  [unwired: 8 in]
              }
              frame True {
                n164 = call "Class Object Construction.vi"("class"=Class_Labels."Valve Controller", "error in"=w392, "classes in"=w396) -> ("error out"=w393:errorcluster, "classes out"=w394:T1)  [unwired: 6 in]
              }
            }
            n165 = call "Device Params Global.vi"("action"=Device_Params_Global."Get Device Connections", "error in"=w375) -> ("error out"=w377:errorcluster, "Device Connections OUT"=w376:T18)  [unwired: 7 in, 1 out]
            n166 = Bundle By Name(cluster=w376, "Valve Controller.Connection"=w374) -> (w379:T18)
            n167 = Select(t=T14."Disabled and Grayed Out" ("Disabled"), s=w374, f=T14."Enabled" ("Disabled")) -> (s? t:f=w384:T14)
            n168 = call "Device Params Global.vi"("action"=Device_Params_Global."Set Device Connections", "error in"=w377, "Device Connections IN"=w379) -> ()  [unwired: 6 in, 3 out]
            n169 = property on="Valve Controller VISA resource name" class="VISAName"("DisabledEnum"=w384) -> (error out=w381:errorcluster)  [unwired: 2 in, 1 out]
          }
          event "Valve Controller VISA resource name": Value Change {
            n170 = event-data() -> ("NewVal"=w398:refnum<visa-resource-name>)  [unwired: 1 in]
            n171 = call "Device Params Global.vi"("action"=Device_Params_Global."Get Device Connections", "error in"=w399) -> ("error out"=w401:errorcluster, "Device Connections OUT"=w400:T18)  [unwired: 7 in, 1 out]
            n172 = Bundle By Name(cluster=w400, "Valve Controller.SMC - INL.VISA resource name"=w398) -> (w403:T18)
            n173 = call "Device Params Global.vi"("action"=Device_Params_Global."Set Device Connections", "error in"=w401, "Device Connections IN"=w403) -> ("error out"=w397:errorcluster)  [unwired: 6 in, 2 out]
          }
        }
      }
    }
  }
  "error out" <- w1
  "Class Objects Out" <- w2
